vi "LatchControlLoop.vi"   [LabVIEW 2014, in "LatchLib.lvlib"]
uses:
  LatchLib.lvlib
  LatchRefs.ctl
  <vilib>/Rock Robotics/WPI/Solenoid/WPI_SolenoidValue.ctl
  <vilib>/Rock Robotics/WPI/Solenoid/WPI_SolenoidSetEnum.vi
types:
  T1 = typedef "LatchLib.lvlib/LatchRefs.ctl" = enum16{"LatchSloenoid", "ContainerSolenoid"}
  T2 = typedef "WPI_SolenoidDevRef.ctl" = cluster{"DevStatus":errorcluster, "Pneumatics Control Module":u8, "Forward Solenoid Channel":T3, "Reverse Solenoid Channel":T3}
  T3 = typedef "WPI_SolenoidChannel.ctl" = enum8{"Solenoid 0", "Solenoid 1", "Solenoid 2", "Solenoid 3", "Solenoid 4", "Solenoid 5", "Solenoid 6", "Solenoid 7", "Invalid"}
  T4 = typedef "WPI_SolenoidValue.ctl" = enum16{"Off", "On", "Forward", "Reverse"}
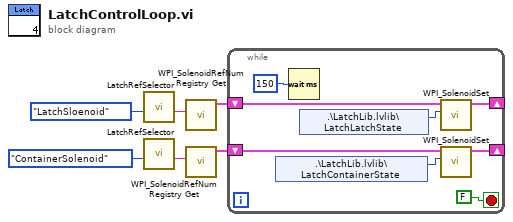
[diagram p0: block diagram]
diagram:
  n1 = call "LatchRefSelector.vi"("Enum"=LatchRefs."LatchSloenoid") -> ("String"=w4:string)  [unwired: 10 in]
  n2 = call "LatchRefSelector.vi"("Enum"=LatchRefs."ContainerSolenoid") -> ("String"=w3:string)  [unwired: 10 in]
  n3 = call <vilib>:"WPI_SolenoidRefNum Registry Get.vi"("refnum name"=w4) -> ("SolenoidDevRef"=w2:T2)  [unwired: 9 in, 1 out]
  n4 = call <vilib>:"WPI_SolenoidRefNum Registry Get.vi"("refnum name"=w3) -> ("SolenoidDevRef"=w1:T2)  [unwired: 9 in, 1 out]
  n5 = while {
    shift-right: [w8] -> _
    shift-left: w2 -> [w9]
    shift-right: [w7] -> _
    shift-left: w1 -> [w10]
    stop <- FALSE stop-if-true
    n6 = shared-variable ".\\LatchLib.lvlib\\LatchContainerState"() -> (w12:T4)  [unwired: 1 in, 1 out]
    n7 = Wait (ms)(milliseconds to wait=u32 150) -> ()  [unwired: 1 out]
    n8 = shared-variable ".\\LatchLib.lvlib\\LatchLatchState"() -> (w13:T4)  [unwired: 1 in, 1 out]
    n9 = call-poly <vilib>:"WPI_SolenoidSet.vi"("Value"=w13, "SolenoidDevRef"=w9) -> ("SolenoidDevRef"=w8:T2)  [unwired: 8 in, 1 out]
    n10 = call-poly <vilib>:"WPI_SolenoidSet.vi"("Value"=w12, "SolenoidDevRef"=w10) -> ("SolenoidDevRef"=w7:T2)  [unwired: 8 in, 1 out]
  }
